vi "Format InstanceStatusSet_LVXML.vi"(8 "error in (no error)":errorcluster, 10 "valueXmlData in":T2, 11 "AWS_EC2 in":refnum<class "AWS_EC2.lvclass">) -> (0 "error out":errorcluster, 2 "Array":T3[](array[typedef]), 3 "AWS_EC2 out":refnum<class "AWS_EC2.lvclass">)   [LabVIEW 2014, in "AWS_EC2.lvlib" / "AWS_EC2.lvclass"]
uses:
  AWS_EC2.lvclass
  EC2 Datatypes/InstanceStatusItemType.ctl
  EC2 Datatypes/InstanceStatusEventType.ctl
  EC2 Datatypes/InstanceStateType.ctl
  EC2 Datatypes/InstanceStatusType.ctl
  EC2 Datatypes/InstanceStatusDetailsSetType.ctl
  lv-xml-parser/r0/trunk/VI Source/EventType.ctl
  lv-xml-parser/r0/trunk/VI Source/LV XML Parser.lvlib
  AWS_EC2.lvlib
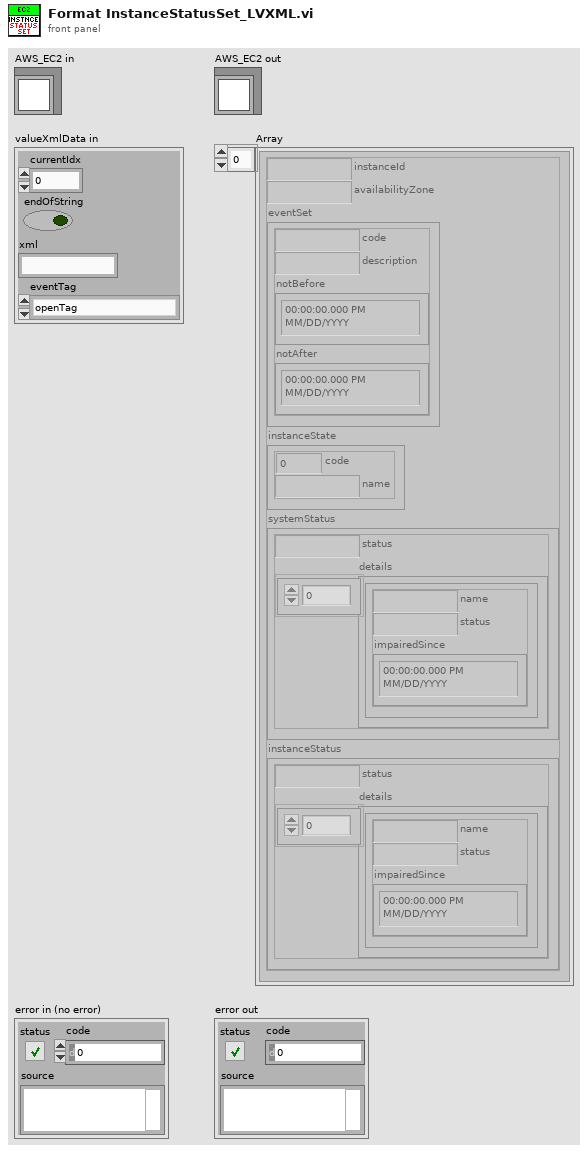
[diagram p1: front panel]
types:
  T1 = typedef "LV XML Parser.lvlib/EventType.ctl" = enum16{"openTag", "endOpenTag", "closeTag", "comment", "endComment", "endOfFile", "attribute", "startXml"}
  T2 = cluster{"currentIdx":i32, "endOfString":bool, "xml":string, "eventTag":T1}
  T3 = typedef "AWS_EC2.lvlib/InstanceStatusItemType.ctl" = cluster{"instanceId":string, "availabilityZone":string, "eventSet":T4, "instanceState":T5, "systemStatus":T6, "instanceStatus":T6}
  T4 = typedef "AWS_EC2.lvlib/InstanceStatusEventType.ctl" = cluster{"code":string, "description":string, "notBefore":timestamp, "notAfter":timestamp}
  T5 = typedef "AWS_EC2.lvlib/InstanceStateType.ctl" = cluster{"code":i16, "name":string}
  T6 = typedef "AWS_EC2.lvlib/InstanceStatusType.ctl" = cluster{"status":string, "details":T7[]}
  T7 = typedef "AWS_EC2.lvlib/InstanceStatusDetailsSetType.ctl" = cluster{"name":string, "status":string, "impairedSince":timestamp}
  T8 = cluster{"namespaceUri":string, "localName":string}
  T9 = cluster{"Attributes":cluster{"localName":string, "namespaceUri":string, "value":string}[], "localName":string, "namespaceUri":string, "valueXmlData":cluster{"currentIdx":i32, "endOfString":bool, "xml":string, "eventTag":T1}}[]
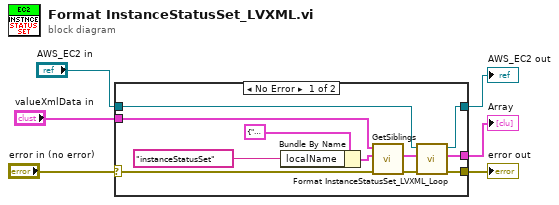
[diagram p0: block diagram]
diagram:
  n1 = case shown="No Error" "error in (no error)" {
    selector: "error in (no error)" -> [w13 w18]
    tunnel: "valueXmlData in" -> [w16 _]
    tunnel: "AWS_EC2 in" -> [w8 w19]
    tunnel: [w7 w19] -> w4
    tunnel: [w11 w18] -> w5
    tunnel: [w12 _] -> w6
    frame No Error {
      n2 = Bundle By Name(cluster=T8 {"namespaceUri"="", "localName"=""} ("limitToTag"), "localName"="instanceStatusSet" ("Tag name")) -> (w14:T8)
      n3 = call "GetSiblings.vi"("error in (no error)"=w13, "limitToTag"=w14, "xmlData"=w16) -> ("error out"=w10:errorcluster, "Siblings"=w9:T9)  [unwired: 7 in]
      n4 = call "Format InstanceStatusSet_LVXML_Loop.vi"("error in (no error)"=w10, "Siblings"=w9, "AWS_EC2 in"=w8) -> ("error out"=w11:errorcluster, "Array"=w12:T3[], "AWS_EC2 out"=w7:refnum<class "AWS_EC2.lvclass">)  [unwired: 6 in]
    }
    frame Error {
    }
  }
  "Array" <- w6
  "error out" <- w5
  "AWS_EC2 out" <- w4
